vi "Get element's ID.vi"(8 "Error in":errorcluster, 11 "GObject in":refnum<vi>) -> (0 "Error out":errorcluster, 3 "ID":string)   [LabVIEW 2019, in "LSS.lvlib"]
doc: "Returns a reference ID for the GObject input. Reference ID contains the name of the object unless the object has no name, in which case a reference number is used.\n\n<b>Inputs:</b>\n<b>GObject in</b> - Reference to the GObject for which a corresponding ID will be found.\n<b>Error In</b> - Error input terminal\n\n<b>Outputs:</b>\n<b>ID</b> - Identification string unique to the control. Usually the label.text property of the control. Exception includes decorations, which use the UID instead.\n<b>Error Out</b> - Error output terminal"
uses:
  LSS.lvlib
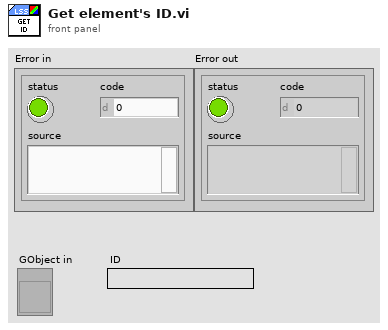
[diagram p1: front panel]
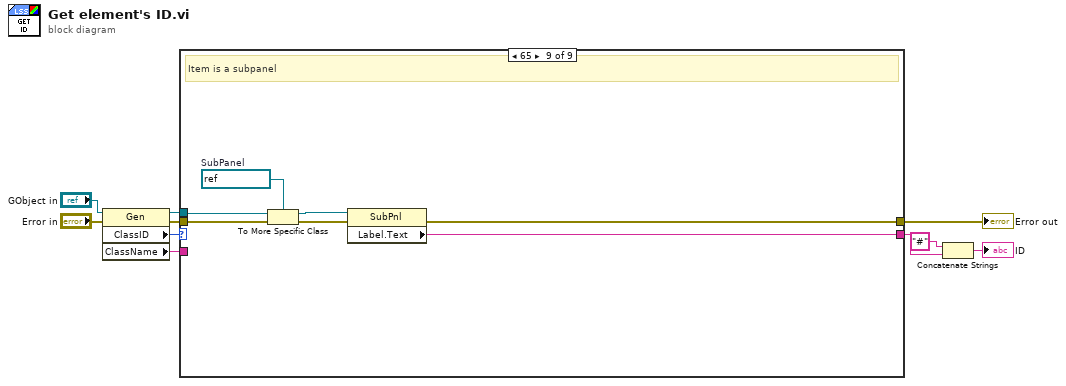
[diagram p0: block diagram]
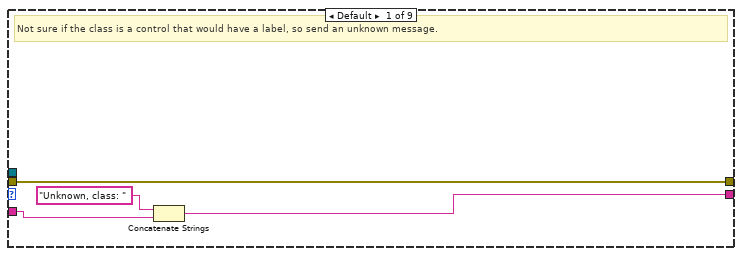
[diagram p2: hidden frame]
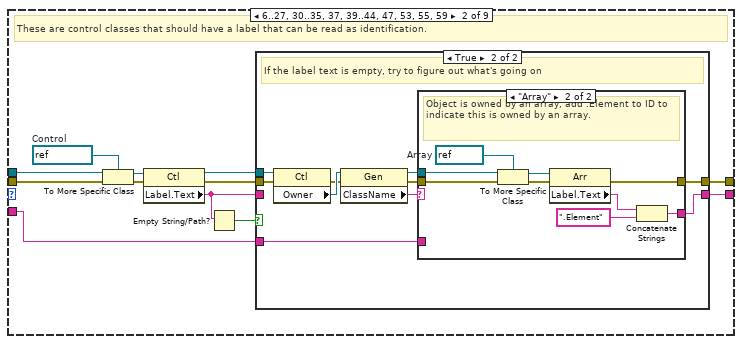
[diagram p3: hidden frame]
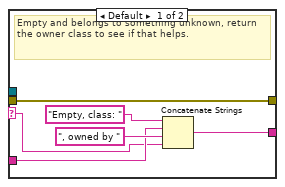
[diagram p5: hidden frame]
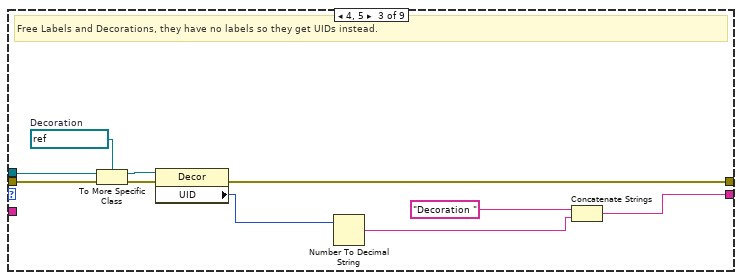
[diagram p6: hidden frame]
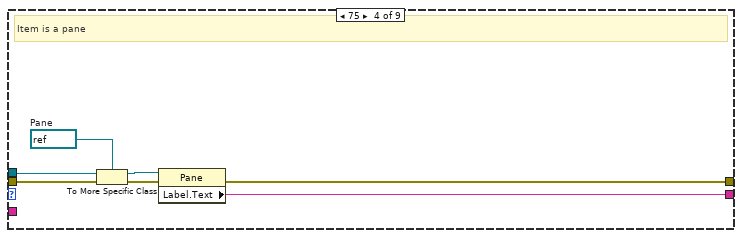
[diagram p7: hidden frame]
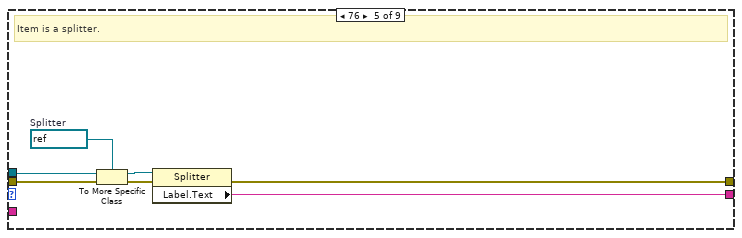
[diagram p8: hidden frame]
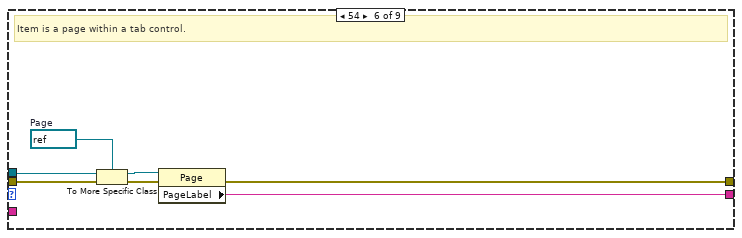
[diagram p9: hidden frame]
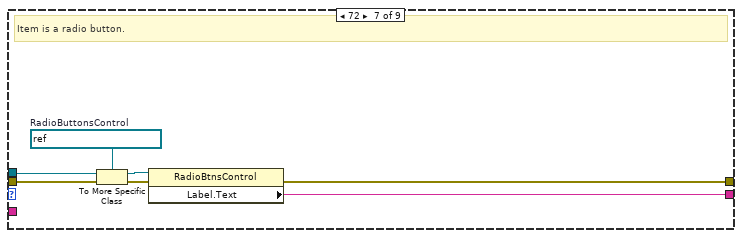
[diagram p10: hidden frame]
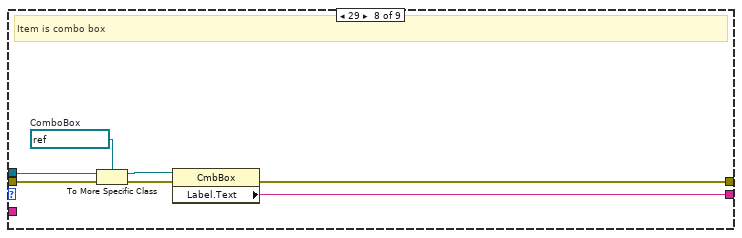
[diagram p11: hidden frame]
diagram:
  n1 = property class="Gen"(reference="GObject in", error in="Error in") -> (reference out=w9:refnum<vi>, error out=w5:errorcluster, "ClassID"=w8:u32, "ClassName"=w3:string)
  n2 = case shown="65" w8 {
    tunnel: [w12 w20 w56 w64 w71 w78 w85 w92 w99] -> w10
    tunnel: w9 -> [_ w25 w62 w69 w76 w83 w90 w97 w104]
    tunnel: w5 -> [w13 w23 w63 w70 w77 w84 w91 w98 w105]
    tunnel: [w13 w15 w58 w65 w72 w79 w86 w93 w100] -> w4
    tunnel: w3 -> [w11 w17 _ _ _ _ _ _ _]
    frame Default {
      # "Not sure if the class is a control that would have a label, so send an unknown message."
      n3 = Concatenate Strings("Unknown, class: ", w11) -> (w12:string)
    }
    frame 6..27, 30..35, 37, 39..44, 47, 53, 55, 59 {
      w26 = refnum<vi> refnum  # Control
      # "These are control classes that should have a label that can be read as identification."
      n4 = To More Specific Class(target class=w26, reference=w25, error in=w23) -> (specific class reference=w24:refnum<vi>, error out=w22:errorcluster)
      n5 = property class="Ctl"(reference=w24, error in=w22) -> (reference out=w18:refnum<vi>, error out=w16:errorcluster, "Label.Text"=w19:string)
      n6 = Empty String/Path?(string/path=w19) -> (empty?=w21:bool)
      n7 = case shown="True" w21 {
        tunnel: [w28 w33] -> w20
        tunnel: w19 -> [w28 _]
        tunnel: w18 -> [_ w38]
        tunnel: w17 -> [_ w35]
        tunnel: w16 -> [w27 w32]
        tunnel: [w27 w29] -> w15
        frame False {
          # "Label has text, use that as the identification."
        }
        frame True {
          # "If the label text is empty, try to figure out what's going on"
          n8 = property class="Ctl"(reference=w38, error in=w32) -> (error out=w31:errorcluster, "Owner"=w37:refnum<vi>)  [unwired: 1 out]
          n9 = property class="Gen"(reference=w37, error in=w31) -> (reference out=w34:refnum<vi>, error out=w30:errorcluster, "ClassName"=w36:string)
          n10 = case shown="\"Array\"" w36 {
            selector: w36 -> [w41 _]
            tunnel: w35 -> [w42 _]
            tunnel: w34 -> [_ w53]
            tunnel: [w40 w48] -> w33
            tunnel: w30 -> [w39 w47]
            tunnel: [w39 w45] -> w29
            frame Default {
              # "Empty and belongs to something unknown, return the owner class to see if that helps."
              n11 = Concatenate Strings("Empty, class: ", w42, ", owned by " ("string"), w41) -> (w40:string)
            }
            frame "Array" {
              w52 = refnum<vi> refnum  # Array
              # "Object is owned by an array, add .Element to ID to indicate this is owned by an array."
              n12 = To More Specific Class(target class=w52, reference=w53, error in=w47) -> (specific class reference=w51:refnum<vi>, error out=w46:errorcluster)
              n13 = property class="Arr"(reference=w51, error in=w46) -> (error out=w45:errorcluster, "Label.Text"=w50:string)  [unwired: 1 out]
              n14 = Concatenate Strings(w50, ".Element" ("string")) -> (w48:string)
            }
          }
        }
      }
    }
    frame 4, 5 {
      w61 = refnum<vi> refnum  # Decoration
      # "Free Labels and Decorations, they have no labels so they get UIDs instead."
      n15 = To More Specific Class(target class=w61, reference=w62, error in=w63) -> (specific class reference=w60:refnum<vi>, error out=w59:errorcluster)
      n16 = property class="Decor"(reference=w60, error in=w59) -> (error out=w58:errorcluster, "UID"=w55:i32)  [unwired: 1 out]
      n17 = Number To Decimal String(number=w55) -> (decimal integer string=w54:string)  [unwired: 1 in]
      n18 = Concatenate Strings("Decoration ", w54) -> (w56:string)
    }
    frame 75 {
      w68 = refnum<vi> refnum  # Pane
      # "Item is a pane"
      n19 = To More Specific Class(target class=w68, reference=w69, error in=w70) -> (specific class reference=w67:refnum<vi>, error out=w66:errorcluster)
      n20 = property class="Pane"(reference=w67, error in=w66) -> (error out=w65:errorcluster, "Label.Text"=w64:string)  [unwired: 1 out]
    }
    frame 76 {
      w75 = refnum<vi> refnum  # Splitter
      # "Item is a splitter."
      n21 = To More Specific Class(target class=w75, reference=w76, error in=w77) -> (specific class reference=w74:refnum<vi>, error out=w73:errorcluster)
      n22 = property class="Splitter"(reference=w74, error in=w73) -> (error out=w72:errorcluster, "Label.Text"=w71:string)  [unwired: 1 out]
    }
    frame 54 {
      w82 = refnum<vi> refnum  # Page
      # "Item is a page within a tab control."
      n23 = To More Specific Class(target class=w82, reference=w83, error in=w84) -> (specific class reference=w81:refnum<vi>, error out=w80:errorcluster)
      n24 = property class="Page"(reference=w81, error in=w80) -> (error out=w79:errorcluster, "PageLabel"=w78:string)  [unwired: 1 out]
    }
    frame 72 {
      w89 = refnum<vi> refnum  # RadioButtonsControl
      # "Item is a radio button."
      n25 = To More Specific Class(target class=w89, reference=w90, error in=w91) -> (specific class reference=w88:refnum<vi>, error out=w87:errorcluster)
      n26 = property class="RadioBtnsControl"(reference=w88, error in=w87) -> (error out=w86:errorcluster, "Label.Text"=w85:string)  [unwired: 1 out]
    }
    frame 29 {
      w96 = refnum<vi> refnum  # ComboBox
      # "Item is combo box"
      n27 = To More Specific Class(target class=w96, reference=w97, error in=w98) -> (specific class reference=w95:refnum<vi>, error out=w94:errorcluster)
      n28 = property class="CmbBox"(reference=w95, error in=w94) -> (error out=w93:errorcluster, "Label.Text"=w92:string)  [unwired: 1 out]
    }
    frame 65 {
      w103 = refnum<vi> refnum  # SubPanel
      # "Item is a subpanel"
      n29 = To More Specific Class(target class=w103, reference=w104, error in=w105) -> (specific class reference=w102:refnum<vi>, error out=w101:errorcluster)
      n30 = property class="SubPnl"(reference=w102, error in=w101) -> (error out=w100:errorcluster, "Label.Text"=w99:string)  [unwired: 1 out]
    }
  }
  "Error out" <- w4
  n31 = Concatenate Strings("#" ("string"), w10) -> (→"ID":string)
